vi "TCP Query.vi"(7 "timeout, ms (5000)":i32=5000, 8 "error in (no error)":errorcluster, 9 "port (53)":u16=53, 10 "address":string="8.8.8.8", 11 "request":T2 {"header"."opcode" items=["Query"=0, "IQuery"=1, "Status"=2, "Notify"=4, "Update"=5, "DSO"=6]; "questions"."class" items=["IN"=1, "CH"=3, "HS"=4, "NONE"=254, "*"=255]; "questions"."type" items=["A"=1, "NS"=2, "MD"=3, "MF"=4, "CNAME"=5, "SOA"=6, "MB"=7, "MG"=8, "MR"=9, "NULL"=10, "WKS"=11, "PTR"=12, "HINFO"=13, "MINFO"=14, "MX"=15, "TXT"=16, "RP"=17, "AFSDB"=18, "X25"=19, "ISDN"=20, "RT"=21, "NSAP"=22, "NSAP-PTR"=23, "SIG"=24, "KEY"=25, "PX"=26, "GPOS"=27, "AAAA"=28, "LOC"=29, "NXT"=30, "EID"=31, "NIMLOC"=32, "SRV"=33, "ATMA"=34, "NAPTR"=35, "KX"=36, "CERT"=37, "A6"=38, "DNAME"=39, "SINK"=40, "OPT"=41, "APL"=42, "DS"=43, "SSHFP"=44, "IPSECKEY"=45, "RRSIG"=46, "NSEC"=47, "DNSKEY"=48, "DHCID"=49, "NSEC3"=50, "NSEC3PARAM"=51, "TLSA"=52, "SMIMEA"=53, "HIP"=55, "NINFO"=56, "RKEY"=57, "TALINK"=58, "CDS"=59, "CDNSKEY"=60, "OPENPGPKEY"=61, "CSYNC"=62, "ZONEMD"=63, "SVCB"=64, "HTTPS"=65, "SPF"=99, "UINFO"=100, "UID"=101, "GID"=102, "UNSPEC"=103, "NID"=104, "L32"=105, "L64"=106, "LP"=107, "EUI48"=108, "EUI64"=109, "TKEY"=249, "TSIG"=250, "IXFR"=251, "AXFR"=252, "MAILB"=253, "MAILA"=254, "*"=255, "URI"=256, "CAA"=257, "AVC"=258, "DOA"=259, "AMTRELAY"=260, "TA"=32768, "DLV"=32769]}) -> (0 "error out":errorcluster)   [LabVIEW 2015, in "PL DNS Client.lvlib"]
doc: "Sends DNS query over TCP to specified <b>address</b> and <b>port</b> and parses received response."
uses:
  PL DNS Client.lvlib
panel:
  out "response":T1 {"header"."response code" items=["NoError"=0, "FormErr"=1, "ServFail"=2, "NXDomain"=3, "NotImp"=4, "Refused"=5, "YXDomain"=6, "YXRRSet"=7, "NXRRSet"=8, "NotAuth"=9, "NotZone"=10, "DSOTYPENI"=11, "BADVERS/BADSIG"=16, "BADKEY"=17, "BADTIME"=18, "BADMODE"=19, "BADNAME"=20, "BADALG"=21, "BADTRUNC"=22, "BADCOOKIE"=23]; "header"."opcode" items=["Query"=0, "IQuery"=1, "Status"=2, "Notify"=4, "Update"=5, "DSO"=6]; "additional records"."class" items=["IN"=1, "CH"=3, "HS"=4]; "additional records"."type" items=["A"=1, "NS"=2, "MD"=3, "MF"=4, "CNAME"=5, "SOA"=6, "MB"=7, "MG"=8, "MR"=9, "NULL"=10, "WKS"=11, "PTR"=12, "HINFO"=13, "MINFO"=14, "MX"=15, "TXT"=16, "RP"=17, "AFSDB"=18, "X25"=19, "ISDN"=20, "RT"=21, "NSAP"=22, "NSAP-PTR"=23, "SIG"=24, "KEY"=25, "PX"=26, "GPOS"=27, "AAAA"=28, "LOC"=29, "NXT"=30, "EID"=31, "NIMLOC"=32, "SRV"=33, "ATMA"=34, "NAPTR"=35, "KX"=36, "CERT"=37, "A6"=38, "DNAME"=39, "SINK"=40, "OPT"=41, "APL"=42, "DS"=43, "SSHFP"=44, "IPSECKEY"=45, "RRSIG"=46, "NSEC"=47, "DNSKEY"=48, "DHCID"=49, "NSEC3"=50, "NSEC3PARAM"=51, "TLSA"=52, "SMIMEA"=53, "HIP"=55, "NINFO"=56, "RKEY"=57, "TALINK"=58, "CDS"=59, "CDNSKEY"=60, "OPENPGPKEY"=61, "CSYNC"=62, "ZONEMD"=63, "SVCB"=64, "HTTPS"=65, "SPF"=99, "UINFO"=100, "UID"=101, "GID"=102, "UNSPEC"=103, "NID"=104, "L32"=105, "L64"=106, "LP"=107, "EUI48"=108, "EUI64"=109, "URI"=256, "CAA"=257, "AVC"=258, "DOA"=259, "AMTRELAY"=260, "TA"=32768, "DLV"=32769]; "authority records"."class" items=["IN"=1, "CH"=3, "HS"=4]; "authority records"."type" items=["A"=1, "NS"=2, "MD"=3, "MF"=4, "CNAME"=5, "SOA"=6, "MB"=7, "MG"=8, "MR"=9, "NULL"=10, "WKS"=11, "PTR"=12, "HINFO"=13, "MINFO"=14, "MX"=15, "TXT"=16, "RP"=17, "AFSDB"=18, "X25"=19, "ISDN"=20, "RT"=21, "NSAP"=22, "NSAP-PTR"=23, "SIG"=24, "KEY"=25, "PX"=26, "GPOS"=27, "AAAA"=28, "LOC"=29, "NXT"=30, "EID"=31, "NIMLOC"=32, "SRV"=33, "ATMA"=34, "NAPTR"=35, "KX"=36, "CERT"=37, "A6"=38, "DNAME"=39, "SINK"=40, "OPT"=41, "APL"=42, "DS"=43, "SSHFP"=44, "IPSECKEY"=45, "RRSIG"=46, "NSEC"=47, "DNSKEY"=48, "DHCID"=49, "NSEC3"=50, "NSEC3PARAM"=51, "TLSA"=52, "SMIMEA"=53, "HIP"=55, "NINFO"=56, "RKEY"=57, "TALINK"=58, "CDS"=59, "CDNSKEY"=60, "OPENPGPKEY"=61, "CSYNC"=62, "ZONEMD"=63, "SVCB"=64, "HTTPS"=65, "SPF"=99, "UINFO"=100, "UID"=101, "GID"=102, "UNSPEC"=103, "NID"=104, "L32"=105, "L64"=106, "LP"=107, "EUI48"=108, "EUI64"=109, "URI"=256, "CAA"=257, "AVC"=258, "DOA"=259, "AMTRELAY"=260, "TA"=32768, "DLV"=32769]; "answers"."class" items=["IN"=1, "CH"=3, "HS"=4]; "answers"."type" items=["A"=1, "NS"=2, "MD"=3, "MF"=4, "CNAME"=5, "SOA"=6, "MB"=7, "MG"=8, "MR"=9, "NULL"=10, "WKS"=11, "PTR"=12, "HINFO"=13, "MINFO"=14, "MX"=15, "TXT"=16, "RP"=17, "AFSDB"=18, "X25"=19, "ISDN"=20, "RT"=21, "NSAP"=22, "NSAP-PTR"=23, "SIG"=24, "KEY"=25, "PX"=26, "GPOS"=27, "AAAA"=28, "LOC"=29, "NXT"=30, "EID"=31, "NIMLOC"=32, "SRV"=33, "ATMA"=34, "NAPTR"=35, "KX"=36, "CERT"=37, "A6"=38, "DNAME"=39, "SINK"=40, "OPT"=41, "APL"=42, "DS"=43, "SSHFP"=44, "IPSECKEY"=45, "RRSIG"=46, "NSEC"=47, "DNSKEY"=48, "DHCID"=49, "NSEC3"=50, "NSEC3PARAM"=51, "TLSA"=52, "SMIMEA"=53, "HIP"=55, "NINFO"=56, "RKEY"=57, "TALINK"=58, "CDS"=59, "CDNSKEY"=60, "OPENPGPKEY"=61, "CSYNC"=62, "ZONEMD"=63, "SVCB"=64, "HTTPS"=65, "SPF"=99, "UINFO"=100, "UID"=101, "GID"=102, "UNSPEC"=103, "NID"=104, "L32"=105, "L64"=106, "LP"=107, "EUI48"=108, "EUI64"=109, "URI"=256, "CAA"=257, "AVC"=258, "DOA"=259, "AMTRELAY"=260, "TA"=32768, "DLV"=32769]}
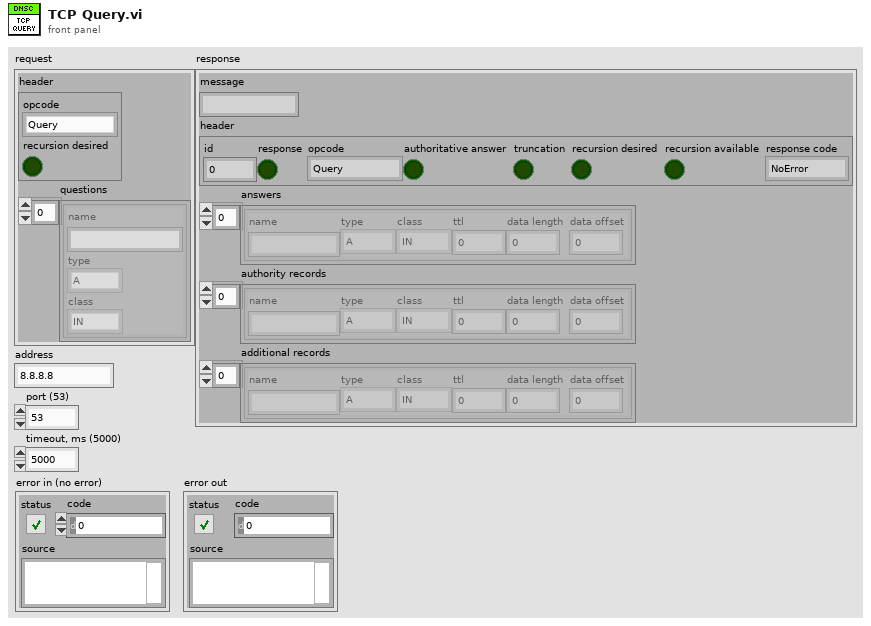
[diagram p1: front panel]
types:
  T1 = cluster{"message":string, "header":cluster{"id":u16, "response":bool, "opcode":u8, "authoritative answer":bool, "truncation":bool, "recursion desired":bool, "recursion available":bool, "response code":u16}, "answers":cluster{"name":string, "type":u16, "class":u16, "ttl":u32, "data length":u16, "data offset":u16}[], "authority records":cluster{"name":string, "type":u16, "class":u16, "ttl":u32, "data length":u16, "data offset":u16}[], "additional records":cluster{"name":string, "type":u16, "class":u16, "ttl":u32, "data length":u16, "data offset":u16}[]}
  T2 = cluster{"header":cluster{"opcode":u8, "recursion desired":bool}, "questions":cluster{"name":string, "type":u16, "class":u16}[]}
  T3 = cluster{"name":string, "type":u16, "class":u16}[]
  T4 = cluster{u16, "opcode":u8, "recursion desired":bool}
  T5 = cluster{cluster{u16, "opcode":u8, "recursion desired":bool}, "questions":cluster{"name":string, "type":u16, "class":u16}[]}
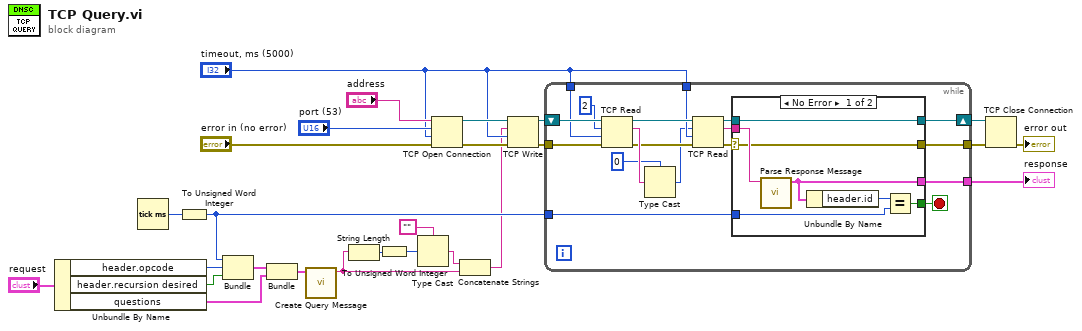
[diagram p0: block diagram]
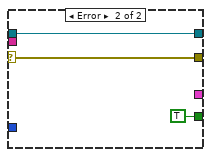
[diagram p2: hidden frame]
diagram:
  n1 = Unbundle By Name("request") -> ("header.opcode"=w25:u8, "header.recursion desired"=w26:bool, "questions"=w22:T3)
  n2 = Tick Count (ms)() -> (millisecond timer value=w5:u32)
  n3 = To Unsigned Word Integer(number=w5) -> (unsigned 16bit integer=w20:u16)
  n4 = Bundle(w20, "opcode"=w25, "recursion desired"=w26) -> (w23:T4)  [unwired: 1 in]
  n5 = Bundle(w23, "questions"=w22) -> (w21:T5)  [unwired: 1 in]
  n6 = call "Create Query Message.vi"("query"=w21) -> ("message"=w7:string)  [unwired: 10 in]
  n7 = String Length(string=w7) -> (length=w6:i32)
  n8 = To Unsigned Word Integer(number=w6) -> (unsigned 16bit integer=w4:u16)
  n9 = Type Cast(type="", x=w4) -> (*(type *) &x=w2:string)
  n10 = TCP Open Connection(address="address", remote port or service name="port (53)", timeout ms (60000)="timeout, ms (5000)", error in (no error)="error in (no error)") -> (connection ID=w13:refnum<k5>, error out=w9:errorcluster)  [unwired: 1 in]
  n11 = Concatenate Strings(w2, w7) -> (w1:string)
  n12 = TCP Write(connection ID=w13, data in=w1, error in (no error)=w9, 9:"timeout, ms (5000)") -> (connection ID out=w15:refnum<k5>, error out=w14:errorcluster)  [unwired: 1 out]
  n13 = while {
    tunnel: w14 -> [w38]
    tunnel: "timeout, ms (5000)" -> [w37]
    shift-right: [w43] -> w17
    shift-left: w15 -> [w39]
    tunnel: [w44] -> w19
    tunnel: [w42] -> w18
    tunnel: w20 -> [w41]
    tunnel: "timeout, ms (5000)" -> [w32]
    stop <- w40 stop-if-true
    n14 = TCP Read(connection ID=w39, bytes to read=2, error in (no error)=w38, 9:w37) -> (connection ID out=w33:refnum<k5>, data out=w35:string, error out=w34:errorcluster)  [unwired: 1 in]
    n15 = Type Cast(type=u16 0, x=w35) -> (*(type *) &x=w31:u16)
    n16 = TCP Read(connection ID=w33, bytes to read=w31, error in (no error)=w34, 9:w32) -> (connection ID out=w28:refnum<k5>, data out=w27:string, error out=w29:errorcluster)  [unwired: 1 in]
    n17 = case shown="No Error" w29 {
      selector: w29 -> [w47 w53]
      tunnel: [w49 _] -> w44
      tunnel: w27 -> [w50 _]
      tunnel: [w48 TRUE] -> w40
      tunnel: w28 -> [w51 w54]
      tunnel: [w51 w54] -> w43
      tunnel: [w47 w53] -> w42
      tunnel: w41 -> [w45 _]
      frame No Error {
        n18 = call "Parse Response Message.vi"("message"=w50) -> ("response"=w49:T1)  [unwired: 10 in]
        n19 = Unbundle By Name(w49) -> ("header.id"=w46:u16)
        n20 = Equal?(x=w46, y=w45) -> (x = y?=w48:bool)
      }
      frame Error {
      }
    }
  }
  "response" <- w19
  n21 = TCP Close Connection(connection ID=w17, error in (no error)=w18) -> (error out=→"error out":errorcluster)  [unwired: 1 in, 1 out]
